vi "Configure UL-DL Pattern.vi"(4 "No Of UL Symbols (4)":i32=4, 5 "No Of UL Slots (4)":i32=4, 6 "No Of DL Symbols (4)":i32=4, 7 "No Of DL Slots (3)":i32=3, 8 "error in (no error)":errorcluster, 9 "Subcarrier Spacing (120 kHz)":T1=1 items=["60 kHz", "120 kHz"], 10 "Instance (1)":T2=1, 11 "VISA resource name":refnum<visa-resource-name>) -> (0 "error out":errorcluster, 3 "VISA resource name out":refnum<visa-resource-name>)   [LabVIEW 2015, in "Rohde&Schwarz CMXP NR FR2 Measurement.lvlib"]
doc: "Configures the UL-DL pattern for the space carrier spacing.\n\nAttribute:\nRSCMXPNRFR2M_ATTR_UL_DL_PATTERN\n\nRemote-control command:\nCONFigure:NRMMw:MEAS<i>:ULDL:PATTern"
uses:
  <instrlib>/Rohde&Schwarz CMXP NR FR2 Measurement/Rohde&Schwarz CMXP NR FR2 Measurement.lvlib
  <instrlib>/Rohde&Schwarz CMXP NR FR2 Measurement/Private/_Instance.ctl
  <instrlib>/Rohde&Schwarz CMXP NR FR2 Measurement/Private/_Subcarrier Spacing.ctl
  <instrlib>/Rohde&Schwarz CMXP NR FR2 Measurement/Private/rsidr_core.llb/rsidr_core.lvlib
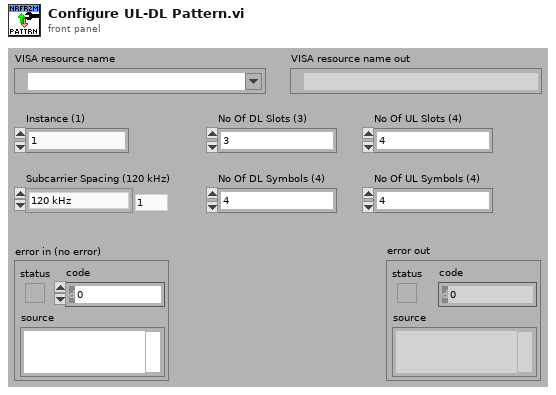
[diagram p1: front panel]
types:
  T1 = typedef "Rohde&Schwarz CMXP NR FR2 Measurement.lvlib/_Subcarrier Spacing.ctl" = i32
  T2 = typedef "Rohde&Schwarz CMXP NR FR2 Measurement.lvlib/_Instance.ctl" = i32
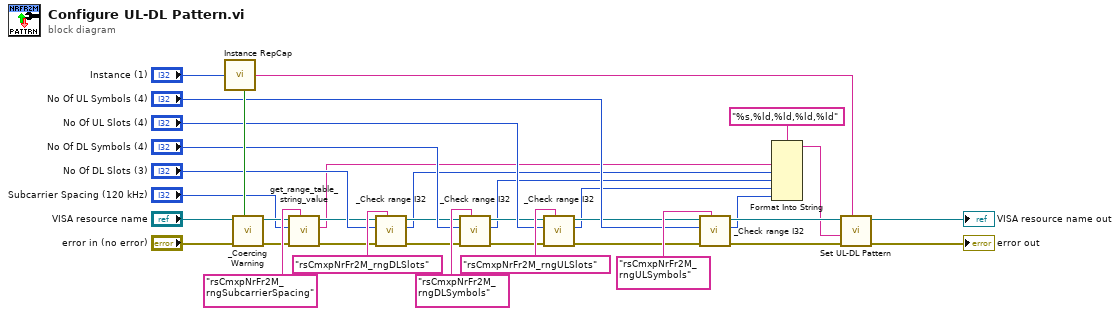
[diagram p0: block diagram]
diagram:
  n1 = call <instrlib>:"Instance RepCap.vi"("Instance In"="Instance (1)") -> ("In Range?"=w35:bool, "RepCap Identifier Out"=w11:string)  [unwired: 1 in]
  n2 = call <instrlib>:"_Coercing Warning.vi"("In Range?"=w35, "error in (no error)"="error in (no error)", "VISA resource name"="VISA resource name") -> ("error out"=w33:errorcluster, "VISA resource name out"=w32:refnum<visa-resource-name>)  [unwired: 7 in]
  n3 = call <instrlib>:"get_range_table_string_value.vi"("Range Table ID in"="rsCmxpNrFr2M_rngSubcarrierSpacing", "error in"=w33, "I32 input"="Subcarrier Spacing (120 kHz)", "VISA resource name"=w32) -> ("error out"=w28:errorcluster, "String Value out"=w7:string, "VISA resource name out"=w27:refnum<visa-resource-name>)  [unwired: 5 in]
  n4 = call <instrlib>:"_Check range I32.vi"("Range Table Identifier"="rsCmxpNrFr2M_rngDLSlots", "error in (no error)"=w28, "I32 Value In"="No Of DL Slots (3)", "VISA resource name"=w27) -> ("error out"=w23:errorcluster, "I32 Value Out"=w6:i32, "VISA resource name out"=w24:refnum<visa-resource-name>)  [unwired: 5 in]
  n5 = call <instrlib>:"_Check range I32.vi"("Range Table Identifier"="rsCmxpNrFr2M_rngDLSymbols", "error in (no error)"=w23, "I32 Value In"="No Of DL Symbols (4)", "VISA resource name"=w24) -> ("error out"=w20:errorcluster, "I32 Value Out"=w5:i32, "VISA resource name out"=w19:refnum<visa-resource-name>)  [unwired: 5 in]
  n6 = call <instrlib>:"_Check range I32.vi"("Range Table Identifier"="rsCmxpNrFr2M_rngULSlots", "error in (no error)"=w20, "I32 Value In"="No Of UL Slots (4)", "VISA resource name"=w19) -> ("error out"=w16:errorcluster, "I32 Value Out"=w4:i32, "VISA resource name out"=w15:refnum<visa-resource-name>)  [unwired: 5 in]
  n7 = call <instrlib>:"_Check range I32.vi"("Range Table Identifier"="rsCmxpNrFr2M_rngULSymbols", "error in (no error)"=w16, "I32 Value In"="No Of UL Symbols (4)", "VISA resource name"=w15) -> ("error out"=w13:errorcluster, "I32 Value Out"=w3:i32, "VISA resource name out"=w12:refnum<visa-resource-name>)  [unwired: 5 in]
  n8 = Format Into String(format string="%s,%ld,%ld,%ld,%ld", w7, w6, w5, w4, w3) -> (resulting string=w1:string)  [unwired: 2 in, 1 out]
  n9 = call "Set UL-DL Pattern"("Repeated Capabilities"=w11, "error in (no error)"=w13, "UL-DL Pattern ()"=w1, "instrument handle"=w12) -> ("error out"=→"error out":errorcluster, "instrument handle out"=→"VISA resource name out":refnum<visa-resource-name>)  [unwired: 6 in]
